vi "Configure Channel.vi"(0 "VISA resource name":refnum<visa-resource-name>, 1 "Trigger Slope (0: Positive)":i32(ring) items=["Positive", "Negative"], 2 "Fixed Trigger Level (1.0)":dbl=1.0, 5 "Channel (0: A)":i32(ring) items=["A", "B", "E"], 7 "Coupling (0: AC)":i32(ring) items=["AC", "DC"], 9 "Attenuation (1.0)":dbl=1.0, 11 "error in (no error)":errorcluster, 12 "Filter (T: On)":bool=TRUE, 13 "Impedance (50 Ohm)":dbl=50.0) -> (4 "VISA resource name out":refnum<visa-resource-name>, 15 "error out":errorcluster)   [LabVIEW 2019, in "Pendulum CNT90.lvlib"]
doc: "Configures the properties of the instrument's channel and specify how you want the counter to couple the input signal for the channel. Sets the scaling factor, input impedance and fixed trigger level."
uses:
  Pendulum CNT90.lvlib
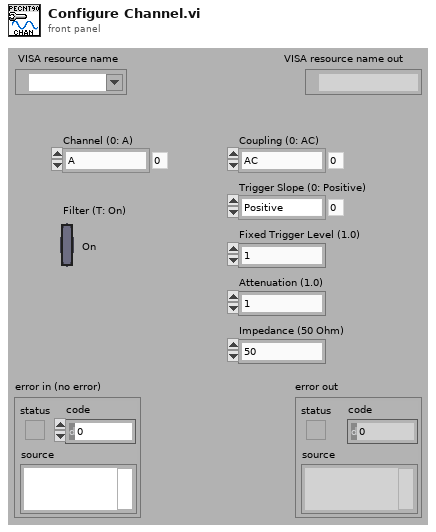
[diagram p1: front panel]
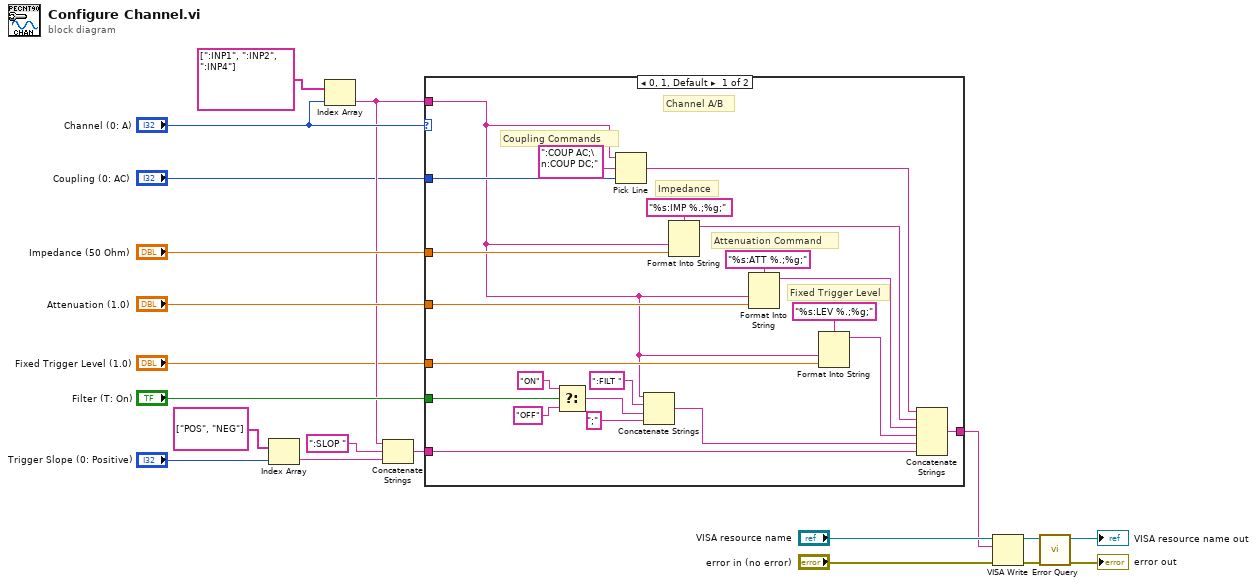
[diagram p0: block diagram]
diagram:
  n1 = Index Array(array=string[] ["POS", "NEG"], index="Trigger Slope (0: Positive)") -> (element=w5:string)
  n2 = Index Array(array=string[] [":INP1", ":INP2", ":INP4"], index="Channel (0: A)") -> (element=w3:string)
  n3 = Concatenate Strings(w3, ":SLOP " ("string"), w5) -> (w4:string)
  n4 = case shown="0, 1, Default" "Channel (0: A)" {
    tunnel: [w39 w43] -> w14
    tunnel: w4 -> [w27 w43]
    tunnel: "Impedance (50 Ohm)" -> [w37 _]
    tunnel: "Attenuation (1.0)" -> [w36 _]
    tunnel: w3 -> [w22 _]
    tunnel: "Filter (T: On)" -> [w31 _]
    tunnel: "Coupling (0: AC)" -> [w25 _]
    tunnel: "Fixed Trigger Level (1.0)" -> [w23 _]
    frame 0, 1, Default {
      # "Channel A/B"
      # "Fixed Trigger Level"
      # "Attenuation Command"
      # "Impedance"
      # "Coupling Commands"
      n5 = Select(t="ON" ("string"), s=w31, f="OFF" ("string")) -> (s? t:f=w29:string)
      n6 = Pick Line(string ("")=w22, multi-line string=":COUP AC;\n:COUP DC;" ("Coupling Commands"), line index=w25) -> (output string=w40:string)
      n7 = Concatenate Strings(w22, ":FILT ", w29, ";" ("string")) -> (w26:string)
      n8 = Format Into String(format string="%s:IMP %.;%g;" ("Impedance"), w22, w37) -> (resulting string=w35:string)  [unwired: 2 in, 1 out]
      n9 = Format Into String(format string="%s:ATT %.;%g;" ("Attenuation Command"), w22, w36) -> (resulting string=w34:string)  [unwired: 2 in, 1 out]
      n10 = Format Into String(format string="%s:LEV %.;%g;" ("Attenuation Command"), w22, w23) -> (resulting string=w21:string)  [unwired: 2 in, 1 out]
      n11 = Concatenate Strings(w40, w35, w34, w21, w26, w27) -> (w39:string)
    }
    frame 2 {
      # "Only Trigger Slope is supported by channel E."
      # "Channel E"
    }
  }
  n12 = VISA Write(VISA resource name="VISA resource name", write buffer=w14, error in (no error)="error in (no error)") -> (VISA resource name out=w16:refnum<visa-resource-name>, error out=w15:errorcluster)  [unwired: 1 out]
  n13 = call "Error Query.vi"("error in (no error)"=w15, "VISA resource name"=w16) -> ("error out"=→"error out":errorcluster, "VISA resource name out"=→"VISA resource name out":refnum<visa-resource-name>)  [unwired: 6 in, 2 out]
